vi "Get Steering Type.vi"(8 "error in (no error)":errorcluster, 11 "differential steering frame in":refnum<class "NI_Robotics_Differential Steering Frame.lvclass">) -> (0 "error out":errorcluster, 2 "steering type":string, 3 "differential steering frame out":refnum<class "NI_Robotics_Differential Steering Frame.lvclass">)   [LabVIEW 2017, in "NI_Robotics_Differential Steering Frame.lvclass"]
uses:
  <vilib>/robotics/Steering/Differential Steering Frame/NI_Robotics_Differential Steering Frame.lvclass
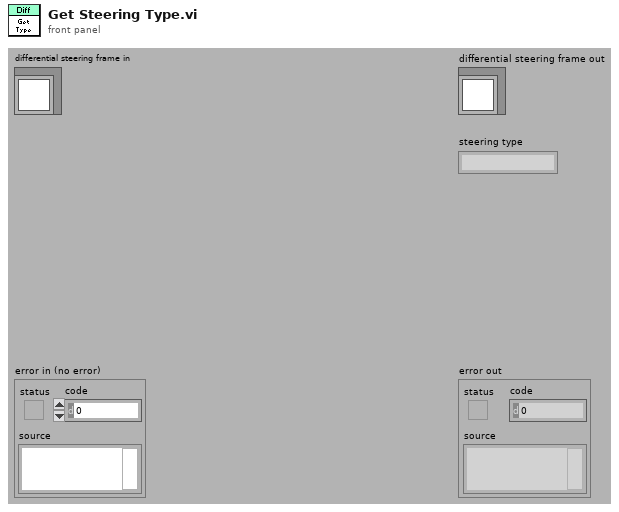
[diagram p1: front panel]
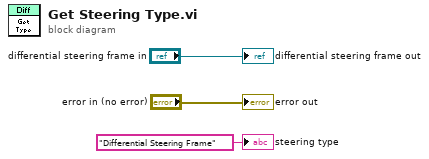
[diagram p0: block diagram]
diagram:
  "error out" <- "error in (no error)"
  "differential steering frame out" <- "differential steering frame in"
  "steering type" <- "Differential Steering Frame" ("Steering Type")
